vi "Firmware Wizard Config.vi"(8 "Error In":errorcluster) -> (0 "Error Out":errorcluster)   [LabVIEW 2013, in "LVH-LINX.lvlib"]
doc: "Allow user to configure settings stored in firmware wizard ini."
uses:
  <vilib>/LabVIEW Hacker/LINX/LVH-LINX.lvlib
  <vilib>/Utility/config.llb/NI_LVConfig.lvlib
  <vilib>/Utility/config.llb/Read Key (Path).vi
  <vilib>/Utility/config.llb/Write Key (Path).vi
panel:
  in  "Cancel Button":bool
  in  "Save Button":bool
  in  "LINX Firmware Builds Base Path":path
  # "Default Location: <LabVIEW>\\vi.lib\\LabVIEW Hacker\\LINX\\Firmware\\Builds"
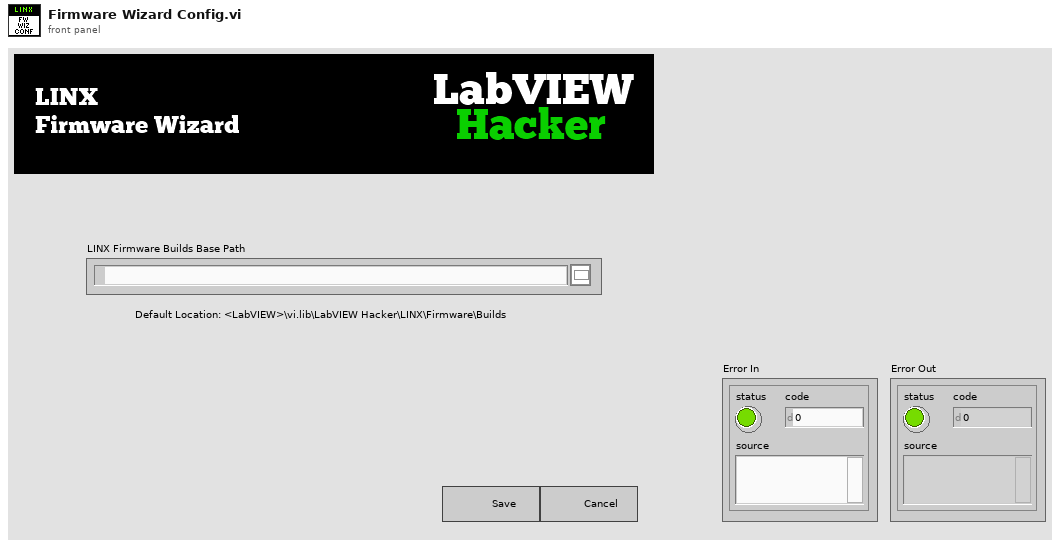
[diagram p1: front panel]
types:
  T1 = typedef "NI_LVConfig.lvlib/Config Data RefNum.ctl" = refnum<k1>
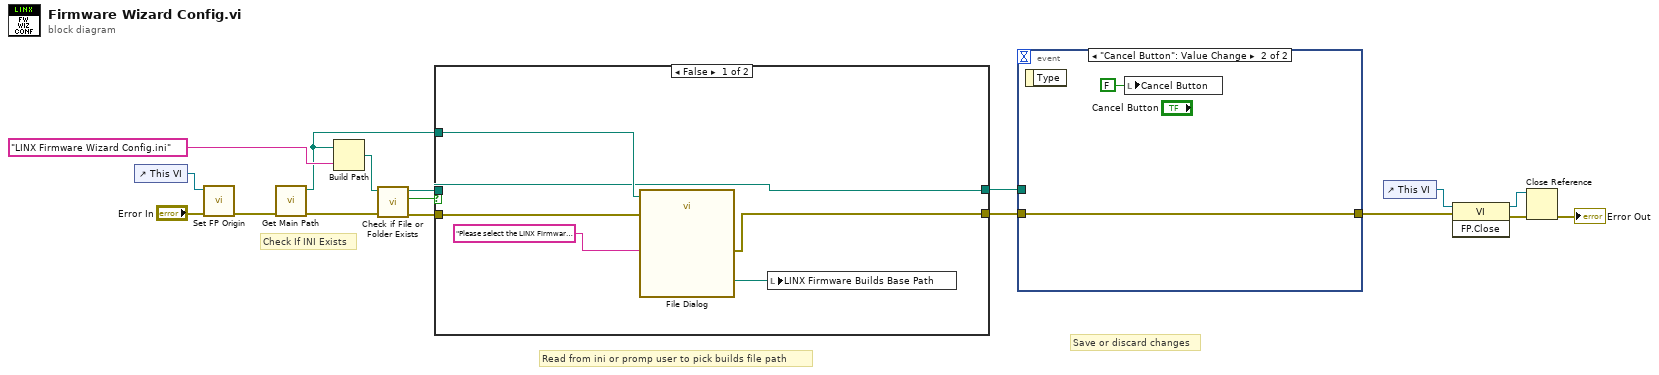
[diagram p0: block diagram]
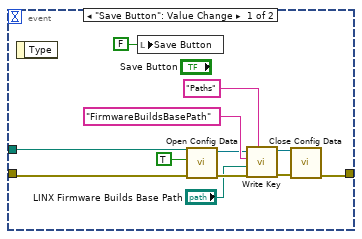
[diagram p2: hidden frame]
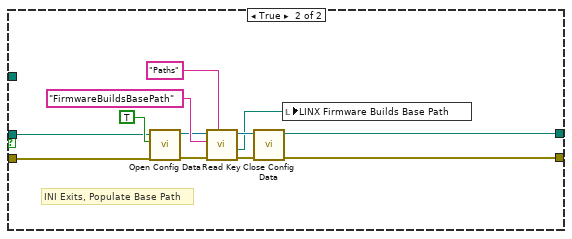
[diagram p3: hidden frame]
diagram:
  # "Save or discard changes"
  # "Read from ini or promp user to pick builds file path"
  # "Check If INI Exists"
  n1 = control-ref of="This VI"() -> (w8:refnum<vi>)
  n2 = call <vilib>:"Set FP Origin.vi"("Error In"="Error In", "VI Ref"=w8) -> ("Error Out"=w1:errorcluster)  [unwired: 9 in]
  n3 = call <vilib>:"Get Main Path.vi"("Error In"=w1) -> ("Error Out"=w16:errorcluster, "Main Dir"=w11:path)  [unwired: 8 in, 1 out]
  n4 = Build Path(base path=w11, name or relative path="LINX Firmware Wizard Config.ini") -> (appended path=w15:path)
  n5 = call <vilib>:"Check if File or Folder Exists.vi"("error in (no error)"=w16, "path"=w15) -> ("error out"=w12:errorcluster, "file or folder exists?"=w13:bool, "dup path"=w14:path)  [unwired: 7 in]
  n6 = case shown="False" w13 {
    tunnel: [w22 w29] -> w10
    tunnel: w14 -> [w20 w27]
    tunnel: w12 -> [w23 w26]
    tunnel: w11 -> [w21 _]
    tunnel: [w20 w25] -> w9
    frame False {
      n7 = call "File Dialog"("start path"=w21, "prompt"="Please select the LINX Firmware builds base directory", "error in"=w23) -> ("selected path"=w19:path, "error out"=w22:errorcluster)  [unwired: 9 in, 2 out]
      n8 = local write "LINX Firmware Builds Base Path"(w19) -> ()
    }
    frame True {
      # "INI Exits, Populate Base Path"
      n9 = call <vilib>:"Open Config Data.vi"("error in (no error)"=w26, "create file if necessary (T)"=TRUE, "configuration file path"=w27) -> ("error out"=w31:errorcluster, "refnum"=w32:T1)  [unwired: 6 in, 1 out]
      n10 = call-poly <vilib>:"Read Key.vi"("section"="Paths", "error in (no error)"=w31, "key"="FirmwareBuildsBasePath", "refnum"=w32) -> ("error out"=w30:errorcluster, "value"=w24:path, "refnum out"=w28:T1)  [unwired: 4 in, 1 out]
      n11 = call <vilib>:"Close Config Data.vi"("error in (no error)"=w30, "refnum"=w28) -> ("error out"=w29:errorcluster, "file path"=w25:path)  [unwired: 8 in]
      n12 = local write "LINX Firmware Builds Base Path"(w24) -> ()
    }
  }
  n13 = event shown="[1] \"Cancel Button\": Value Change" {
    selector: _ -> [_ _]
    dyn-events: _ -> [_ _]
    timeout: _ -> [_ _]
    tunnel: w10 -> [w44 w48]
    tunnel: [w37 w48] -> w3
    tunnel: w9 -> [w40 _]
    event "Save Button": Value Change {
      n14 = event-data() -> ()  [unwired: 1 in, 1 out]
      n15 = local write "Save Button"(FALSE ("Save Button")) -> ()
      n16 = call <vilib>:"Open Config Data.vi"("error in (no error)"=w44, "create file if necessary (T)"=TRUE, "configuration file path"=w40) -> ("error out"=w43:errorcluster, "refnum"=w39:T1)  [unwired: 6 in, 1 out]
      n17 = call-poly <vilib>:"Write Key.vi"("section"="Paths", "error in (no error)"=w43, "value"="LINX Firmware Builds Base Path", "key"="FirmwareBuildsBasePath", "refnum"=w39) -> ("error out"=w45:errorcluster, "refnum out"=w38:T1)  [unwired: 4 in, 1 out]
      n18 = call <vilib>:"Close Config Data.vi"("error in (no error)"=w45, "refnum"=w38) -> ("error out"=w37:errorcluster)  [unwired: 8 in, 1 out]
    }
    event "Cancel Button": Value Change {
      n19 = event-data() -> ()  [unwired: 1 in, 1 out]
      n20 = local write "Cancel Button"(FALSE ("Cancel Button")) -> ()
    }
  }
  n21 = control-ref of="This VI"() -> (w4:refnum<vi>)
  n22 = invoke class="VI" method="FP.Close"(reference=w4, error in=w3) -> (reference out=w6:refnum<vi>, error out=w5:errorcluster)  [unwired: 1 in, 1 out]
  n23 = Close Reference(reference=w6, error in (no error)=w5) -> (error out=→"Error Out":errorcluster)
